vi "Test - Draw Line Algorithm Comparison.vi"() -> ()   [LabVIEW 2022 SP3, in "Raster.lvlib"]
uses:
  Raster.lvlib
  Rectangle Dimensions.ctl
  Point 2D (I32).ctl
  <vilib>/numeric/Random Number (Range) U64.vi
  5ddc0be9-1862-4ec3-be50-f9cb0509fb6a.vi
  908fe56b-1897-4fa8-9649-fb77c4eaa338.vi
  4d47050f-d93e-41b0-9249-b91c5f7c868d.vi
  9a67d9ed-7d21-4ca8-b675-744834f4f57d.vi
  <vilib>/Analysis/baseanly.llb/Mean (DBL).vi
  <vilib>/numeric/sub_Random U32.vi
  <vilib>/Utility/High Resolution Relative Seconds.vi
  <vilib>/Analysis/NI_AALBase.lvlib
panel:
  out "Array":bool[](array[boolean])
  out "Numeric":i32
  out "x = y?":bool
  out "v2 mean":dbl format="%.1p"
  out "v1 mean":dbl format="%.1p"
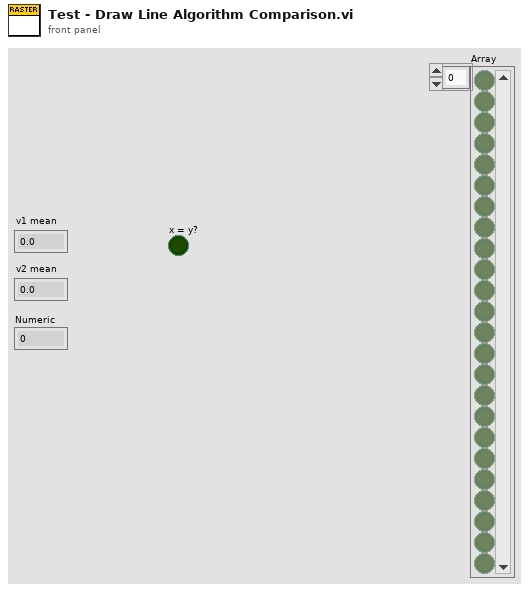
[diagram p1: front panel]
types:
  T1 = typedef "Raster.lvlib/Rectangle Dimensions.ctl" = cluster{"Width":u32, "Height":u32}
  T2 = typedef "Raster.lvlib/Point 2D (I32).ctl" = cluster{"x":i32, "y":i32}
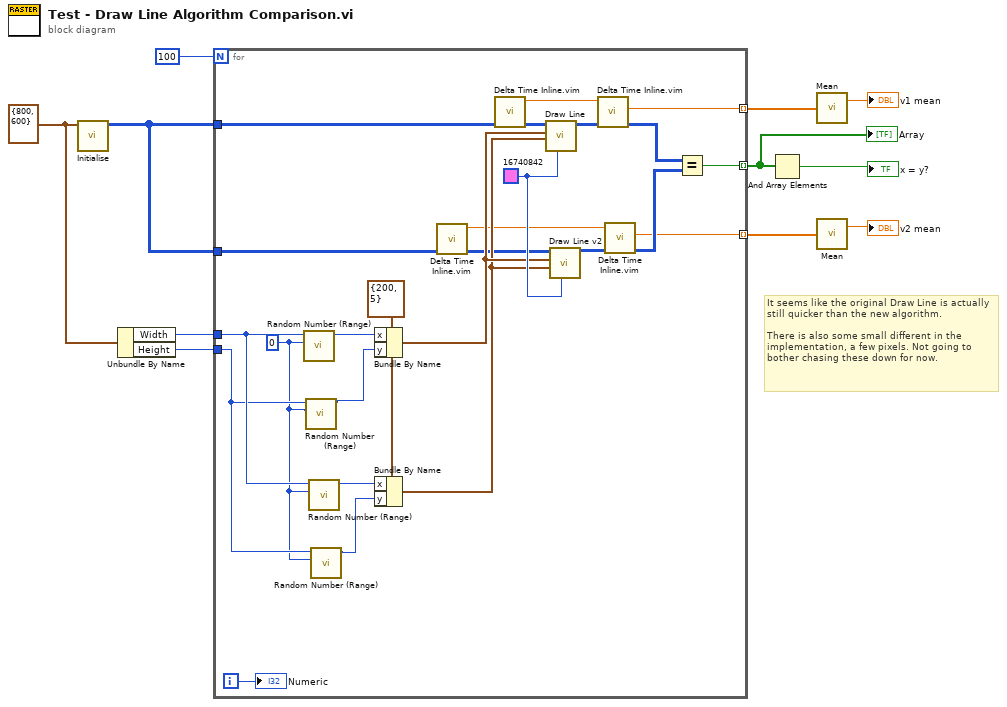
[diagram p0: block diagram]
diagram:
  w3 = T1 {"Width"=800, "Height"=600} ("Screen Dimensions")
  # "It seems like the original Draw Line is actually still quicker than the new algorithm.\n\nThere is also some small different in the implementation, a few pixels. Not going to bother chasing these down for now."
  n1 = call "Initialise.vi"("Screen Dimensions"=w3) -> ("Pixel Data out"=w7:u32[][])  [unwired: 10 in]
  n2 = Unbundle By Name(w3) -> ("Width"=w2:u32, "Height"=w1:u32)
  n3 = for {
    N: 100 -> [_]
    tunnel: w7 -> [w22]
    tunnel: [w25] -> w5 mode=indexing
    tunnel: [w19] -> w8 mode=indexing
    tunnel: w7 -> [w16]
    tunnel: [w12] -> w6 mode=indexing
    tunnel: w2 -> [w32]
    tunnel: w1 -> [w31]
    i -> [w24]
    w30 = u64 0 ("lower bound (0)")
    w33 = T2 {"x"=200, "y"=5} ("Point 1")
    w36 = u32 16740842 ("Colour")
    n4 = call-poly <vilib>:"Random Number (Range).vi"("lower bound (0)"=w30, "upper bound (100)"=w32) -> ("number"=w35:u64)  [unwired: 9 in]
    n5 = call-poly <vilib>:"Random Number (Range).vi"("lower bound (0)"=w30, "upper bound (100)"=w31) -> ("number"=w34:u64)  [unwired: 9 in]
    n6 = call-poly <vilib>:"Random Number (Range).vi"("lower bound (0)"=w30, "upper bound (100)"=w32) -> ("number"=w29:u64)  [unwired: 9 in]
    n7 = call-poly <vilib>:"Random Number (Range).vi"("lower bound (0)"=w30, "upper bound (100)"=w31) -> ("number"=w28:u64)  [unwired: 9 in]
    n8 = Bundle By Name(cluster=w33, "x"=w35, "y"=w34) -> (w27:T2)
    n9 = Bundle By Name(cluster=w33, "x"=w29, "y"=w28) -> (w26:T2)
    n10 = call "Delta Time Inline.vim"("value in"=w16) -> ("value out"=w17:u32[][], "Relative Seconds out [s]"=w13:dbl)  [unwired: 8 in, 1 out]
    n11 = call "Delta Time Inline.vim"("value in"=w22) -> ("value out"=w23:u32[][], "Relative Seconds out [s]"=w20:dbl)  [unwired: 8 in, 1 out]
    n12 = call "Draw Line.vi"("Colour"=w36, "Point 2"=w26, "Point 1"=w27, "Pixel Data in"=w23) -> ("Pixel Data out"=w21:u32[][])  [unwired: 7 in]
    n13 = call "Draw Line v2.vi"("Colour"=w36, "Point 2"=w26, "Point 1"=w27, "Pixel Data in"=w17) -> ("Pixel Data out"=w15:u32[][])  [unwired: 7 in]
    n14 = call "Delta Time Inline.vim"("value in"=w21, "Relative Seconds in [s]"=w20) -> ("value out"=w18:u32[][], "Delta Time [s]"=w19:dbl)  [unwired: 7 in, 1 out]
    n15 = call "Delta Time Inline.vim"("value in"=w15, "Relative Seconds in [s]"=w13) -> ("value out"=w14:u32[][], "Delta Time [s]"=w12:dbl)  [unwired: 7 in, 1 out]
    n16 = Equal?(x=w18, y=w14) -> (x = y?=w25:bool)
    "Numeric" <- w24
  }
  "Array" <- w5
  n17 = And Array Elements(Boolean array=w5) -> (logical AND=→"x = y?":bool)
  n18 = call-poly <vilib>:"Mean.vi"("X"=w8) -> ("mean"=→"v1 mean":dbl)  [unwired: 1 out]
  n19 = call-poly <vilib>:"Mean.vi"("X"=w6) -> ("mean"=→"v2 mean":dbl)  [unwired: 1 out]
